vi "Keithley DMM7510 Buffer Actual End.vi"(6 "Timeout (10000 ms)":i32=10000 format="%#.6g", 8 "error in (no error)":errorcluster, 10 "Buffer Name (defbuffer1)":string="defbuffer1", 11 "VISA resource name":refnum<visa-resource-name>) -> (0 "error out":errorcluster, 2 "Actual End":i32, 3 "VISA resource name out":refnum<visa-resource-name>)   [LabVIEW 2016]
uses:
  Keithley DMM7510.lvlib
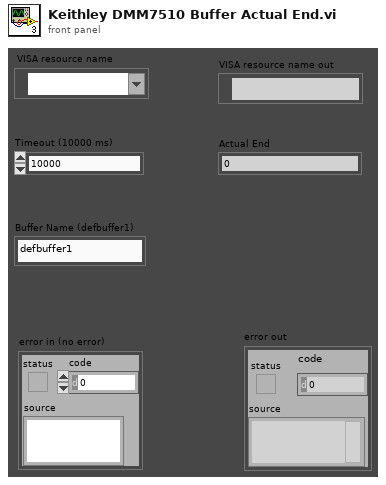
[diagram p1: front panel]
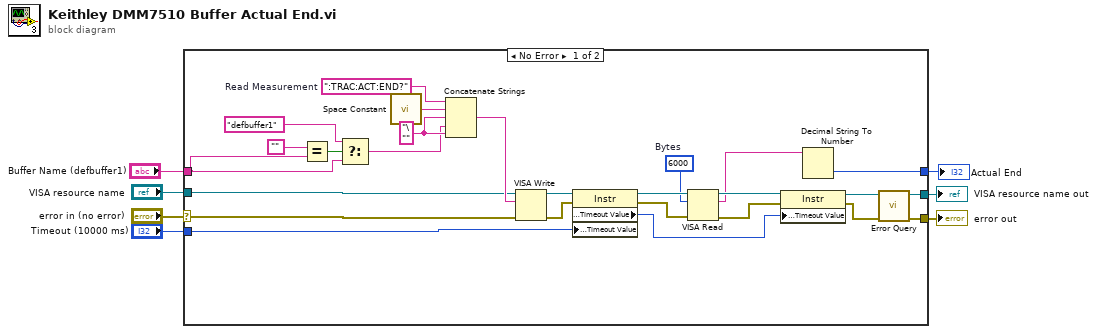
[diagram p0: block diagram]
diagram:
  n1 = case shown="No Error" "error in (no error)" {
    selector: "error in (no error)" -> [w14 w35]
    tunnel: [w33 w35] -> w7
    tunnel: "Buffer Name (defbuffer1)" -> [w21 _]
    tunnel: "VISA resource name" -> [w15 w34]
    tunnel: "Timeout (10000 ms)" -> [w13 _]
    tunnel: [w12 w34] -> w2
    tunnel: [w8 _] -> w1
    frame No Error {
      w19 = "\""
      w16 = ":TRAC:ACT:END?"  # Read Measurement
      w25 = u32 6000  # Bytes
      n2 = Equal?(x="", y=w21) -> (x = y?=w22:bool)
      n3 = Select(t="defbuffer1", s=w22, f=w21) -> (s? t:f=w18:string)
      n4 = call <vilib>:"Space Constant.vi"() -> ("String"=w17:string)
      n5 = Concatenate Strings(w16, w17, w19, w18, w19) -> (w32:string)
      n6 = VISA Write(VISA resource name=w15, write buffer=w32, error in (no error)=w14) -> (VISA resource name out=w24:refnum<visa-resource-name>, error out=w31:errorcluster)  [unwired: 1 out]
      n7 = property class="Instr"(reference=w24, error in=w31, "General Settings:Timeout Value"=w13) -> (reference out=w30:refnum<visa-resource-name>, error out=w29:errorcluster, "General Settings:Timeout Value"=w26:u32)
      n8 = VISA Read(VISA resource name=w30, byte count=w25, error in (no error)=w29) -> (VISA resource name out=w28:refnum<visa-resource-name>, read buffer=w9:string, error out=w27:errorcluster)  [unwired: 1 out]
      n9 = property class="Instr"(reference=w28, error in=w27, "General Settings:Timeout Value"=w26) -> (reference out=w11:refnum<visa-resource-name>, error out=w10:errorcluster)
      n10 = Decimal String To Number(string=w9) -> (number=w8:i32)  [unwired: 2 in, 1 out]
      n11 = call "Error Query.vi"("error in (no error)"=w10, "VISA resource name"=w11) -> ("error out"=w33:errorcluster, "VISA resource name out"=w12:refnum<visa-resource-name>)  [unwired: 8 out]
    }
    frame Error {
    }
  }
  "error out" <- w7
  "VISA resource name out" <- w2
  "Actual End" <- w1
